vi "Keep Average.vi"(7 "Reset(F)":bool, 11 "Value":dbl) -> (3 "Average":dbl)   [LabVIEW 2017]
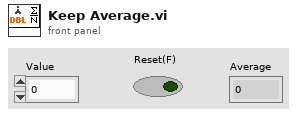
[diagram p1: front panel]
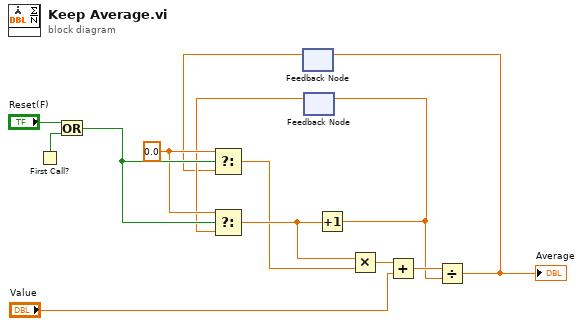
[diagram p0: block diagram]
diagram:
  w10 = 0.0 ("t")
  n1 = First Call?() -> (First Call?: T/F=w12:bool)
  n2 = Or(x="Reset(F)", y=w12) -> (x .or. y?=w11:bool)
  n3 = feedback #1() -> (w2:dbl)  [unwired: 1 in]
  n4 = Select(t=w10, s=w11, f=w2) -> (s? t:f=w7:dbl)
  n5 = feedback #2() -> (w9:dbl)  [unwired: 1 in]
  n6 = Select(t=w10, s=w11, f=w9) -> (s? t:f=w8:dbl)
  n7 = Increment(x=w8) -> (x+1=w3:dbl)
  n8 = feedback-in #2(w3) -> ()
  n9 = Multiply(x=w8, y=w7) -> (x*y=w6:dbl)
  n10 = Add(x=w6, y="Value") -> (x+y=w4:dbl)
  n11 = Divide(x=w4, y=w3) -> (x/y=w1:dbl)
  "Average" <- w1
  n12 = feedback-in #1(w1) -> ()
